vi "Create Test Configuration.vi"() -> (0 "error out":errorcluster, 1 "channel names":string[](array[string]), 2 "Lines":T1[](array[typedef]), 3 "Module Configuration":refnum<class "Shared Memory configuration.lvclass">, 4 "Channels":refnum<class "TBM channel.lvclass">[](array[class]), 5 "instance identifier":string)   [LabVIEW 2013, in "Shared Memory tests.lvlib"]
doc: "This VI creates a standard test configuration for other unit tests. It currently creates and adds one line with every datatype to the module configuration."
uses:
  Shared Memory tests.lvlib
  module/configuration/Shared Memory configuration.lvclass
  module/configuration/Line.ctl
  <vilib>/NI/Tag Bus Module Framework/channel/TBM channel.lvclass
  module/configuration/Shared Memory configuration.lvclass/Shared Memory configuration.ctl
  module/configuration/Write Input File String.vi
  module/configuration/Write Output File String.vi
  module/configuration/Write C Header File Directory.vi
  module/configuration/Write c header file string.vi
  module/configuration/Write sync struct name.vi
  <vilib>/NI/Configuration Framework/serializable configuration/NISE_CEF_serializable configuration.lvclass
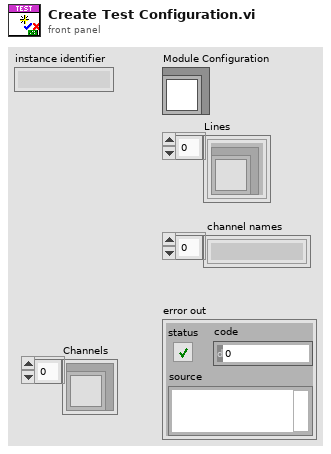
[diagram p1: front panel]
types:
  T1 = typedef "Shared Memory configuration.lvclass/Line.ctl" = cluster{"channel":refnum<class "TBM channel.lvclass">}
  T2 = typedef "tag bus.lvlib/tag descriptor.lvclass/Data Type.ctl" = enum16{"Double", "Single", "I64", "I32", "I16", "I8", "U64", "U32", "U16", "U8", "Boolean", "String", "Array of Double", "Array of Single", "Array of I64", "Array of I32", "Array of I16", "Array of I8", "Array of U64", "Array of U32", "Array of U16", "Array of U8", "Array of Boolean", "Array of String"}
  T3 = typedef "TBM channel.lvclass/channel classification.ctl" = enum16{"input data", "output data", "processing parameter", "processing result"}
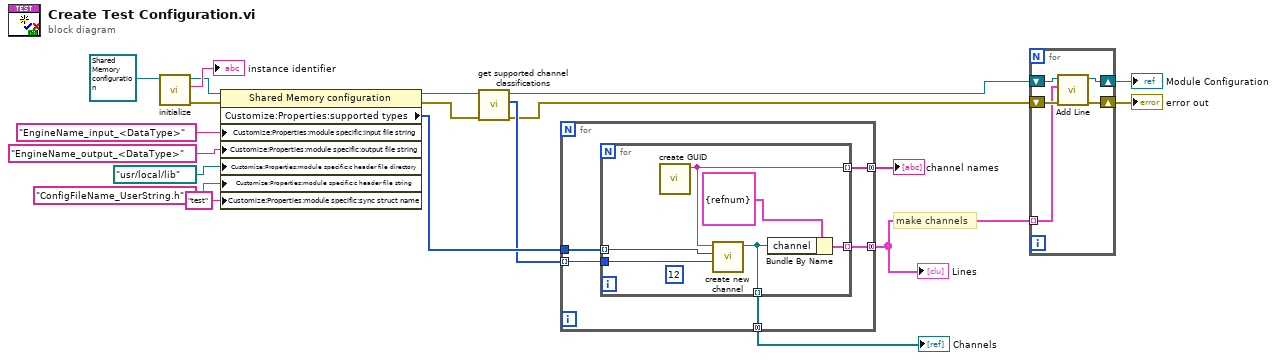
[diagram p0: block diagram]
diagram:
  # "make channels"
  n1 = call <vilib>:"initialize.vi"("configuration in"=refnum<class "Shared Memory configuration.lvclass"> refnum ("tag bus configurable plugin module configuration")) -> ("error out"=w18:errorcluster, "identifier"=→"instance identifier":string, "configuration out"=w16:refnum<class "Shared Memory configuration.lvclass">)  [unwired: 8 in]
  n2 = property class="Shared Memory configuration"(reference=w16, error in=w18, "Customize:Properties:module specific:input file string"="EngineName_input_<DataType>", "Customize:Properties:module specific:output file string"="EngineName_output_<DataType>", "Customize:Properties:module specific:c header file directory"=path "/usr/local/lib" ("c header file directory"), "Customize:Properties:module specific:c header file string"="ConfigFileName_UserString.h" ("name string"), "Customize:Properties:module specific:sync struct name"="test" ("sync struct name")) -> (reference out=w6:refnum<class "Shared Memory configuration.lvclass">, error out=w3:errorcluster, "Customize:Properties:supported types"=w13:T2[])
  n3 = call-dynamic "get supported channel classifications.vi"("error in"=w3, "module configuration in"=w6) -> ("error out"=w2:errorcluster, "supported classes"=w4:T3[], "module configuration out"=w5:refnum<class "Shared Memory configuration.lvclass">)  [unwired: 7 in]
  n4 = for {
    tunnel: w4 -> [w25] mode=indexing
    tunnel: [w23] -> w15 mode=concatenating
    tunnel: w13 -> [w24]
    tunnel: [w22] -> w17 mode=concatenating
    tunnel: [w21] -> w12 mode=concatenating
    n5 = for {
      tunnel: w25 -> [w31]
      tunnel: [w27] -> w23 mode=indexing
      tunnel: w24 -> [w30] mode=indexing
      tunnel: [w29] -> w22 mode=indexing
      tunnel: [w26] -> w21 mode=indexing
      (unwired) 12
      n6 = call <vilib>:"create GUID.vi"() -> ("uuid"=w29:string)  [unwired: 10 in, 1 out]
      n7 = call <vilib>:"create new channel.vi"("channel classification"=w31, "data type"=w30, "channel name"=w29) -> ("channel"=w26:refnum<class "TBM channel.lvclass">)  [unwired: 8 in]
      n8 = Bundle By Name(cluster=T1 {"channel"=refnum} ("Line"), "channel"=w26) -> (w27:T1)
    }
  }
  "channel names" <- w17
  "Lines" <- w15
  "Channels" <- w12
  n9 = for {
    tunnel: w15 -> [w32] mode=indexing
    shift-right: [w35] -> w14
    shift-left: w5 -> [w36]
    shift-right: [w33] -> w20
    shift-left: w2 -> [w34]
    n10 = call "Add Line.vi"("error in"=w34, "Line"=w32, "Shared Memory configuration in"=w36) -> ("error out"=w33:errorcluster, "Shared Memory configuration out"=w35:refnum<class "Shared Memory configuration.lvclass">)  [unwired: 6 in, 1 out]
  }
  "error out" <- w20
  "Module Configuration" <- w14
